vi "0x2 RIO-OCU command receive.vi"(11 "Manual Override Reader In":refnum<class "NetworkStreamReader.lvclass">) -> (3 "Manual Override Reader Out":refnum<class "NetworkStreamReader.lvclass">)   [LabVIEW 2011]
doc: "Gets commands from the OCU and sends them out to the rest of the code on the RIO using the globals."
uses:
  0x2 Classes/NetworkStreams/Reader/NetworkStreamReader.lvclass
  0x2 Typedefs/ocuCommands.ctl
  0x2 Typedefs/manual override.ctl
  2-Think/2 Typedefs/setpoints to boat.ctl
  2-Think/2 Typedefs/sail setpt.ctl
  2-Think/2 Typedefs/rudder angle.ctl
  0x2 Typedefs/ocuMessage.ctl
  2-Think/2 Classes/Waypoint/Waypoint.lvclass
  2-Think/2 Typedefs/UTM Circle.ctl
  2-Think/2 Classes/Missions/GenericMission/GenericMission.lvclass
  0x2 Typedefs/Current Waypoint.ctl
  0x2 Typedefs/Control values.ctl
  2-Think/2 Typedefs/Goodness Weightings.ctl
  2-Think/2 Typedefs/PI Constants.ctl
  2-Think/2 Typedefs/Apparent Wind Mode.ctl
  0x2 Typedefs/Sail Setting Tuning.ctl
  2-Think/2 Globals/2 Global.vi
  2-Think/2 Globals/2 TuningConstants.vi
  2-Think/2 Globals/2 Message Logger.vi
  2-Think/2 Classes/MissionQueue/MissionQueue.lvclass
  2-Think/2 Classes/Logger/Logger.lvclass
panel:
  out "Latest OCU Command":T1
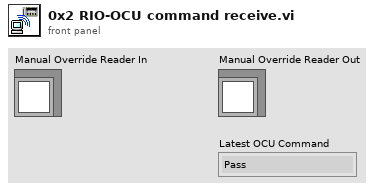
[diagram p1: front panel]
types:
  T1 = typedef "ocuCommands.ctl" = enum16{"Pass", "Send override", "Add waypoint", "Set waypoint number", "Stop", "Add Mission", "Reset Missions/Waypts", "Edit Control Values", "Add Global No-Sail", "Log Message"}
  T2 = typedef "manual override.ctl" = cluster{"Override Active Rudder":bool, "Setpoints":T3, "Override Active Sail":bool}
  T3 = typedef "setpoints to boat.ctl" = cluster{"Sail Position":T4, "Rudder Angle":T5}
  T4 = typedef "sail setpt.ctl" = dbl
  T5 = typedef "rudder angle.ctl" = dbl
  T6 = typedef "ocuMessage.ctl" = cluster{"OCU Command":T1, "Data":variant}
  T7 = typedef "UTM Circle.ctl" = cluster{"UTM Zone":dbl, "Hemisphere":enum16{"North", "South"}, "East":dbl, "North":dbl, "Radius":dbl}
  T8 = typedef "Current Waypoint.ctl" = i32
  T9 = typedef "Control values.ctl" = cluster{"Goodness Weightings":T10, "PI Constants":T11, "No Sail Zone\nTuning Quotient":dbl, "Heading Change Wind Adjustment":dbl, "Waypoint Tuning Quotient":dbl, "Apparent Wind Mode":T12, "RP Autonomous":bool, "Let Sail Out on Windcross":bool, "Shift Goal for currents":bool, "Round Buoy Safety":dbl, "Sail Setting Options":T13, "Defilter Wind Data":bool, "Irons Range":dbl, "Convincing Range":dbl, "Run Range":dbl, "Force tack attempt?":bool, "Minimum\ntack try\ntime?":dbl}
  T10 = typedef "Goodness Weightings.ctl" = cluster{"Target Importance":dbl, "No Sail Importance":dbl, "Change Importance":dbl, "Pure Waypoint \nImportance":dbl, "Pure Wind \nImportance":dbl}
  T11 = typedef "PI Constants.ctl" = cluster{"Proportional Gain":dbl, "Integral Time":dbl, "Derivative Time":dbl}
  T12 = typedef "Apparent Wind Mode.ctl" = cluster{"Desired Apparent\nWind Direction":dbl, "On":bool}
  T13 = typedef "Sail Setting Tuning.ctl" = cluster{"Linear\nMode":bool, "Sails Full In Point":dbl, "Sails Full Out Point":dbl}
  T14 = typedef "Waypoints List.ctl" = refnum<class "Waypoint.lvclass">[]
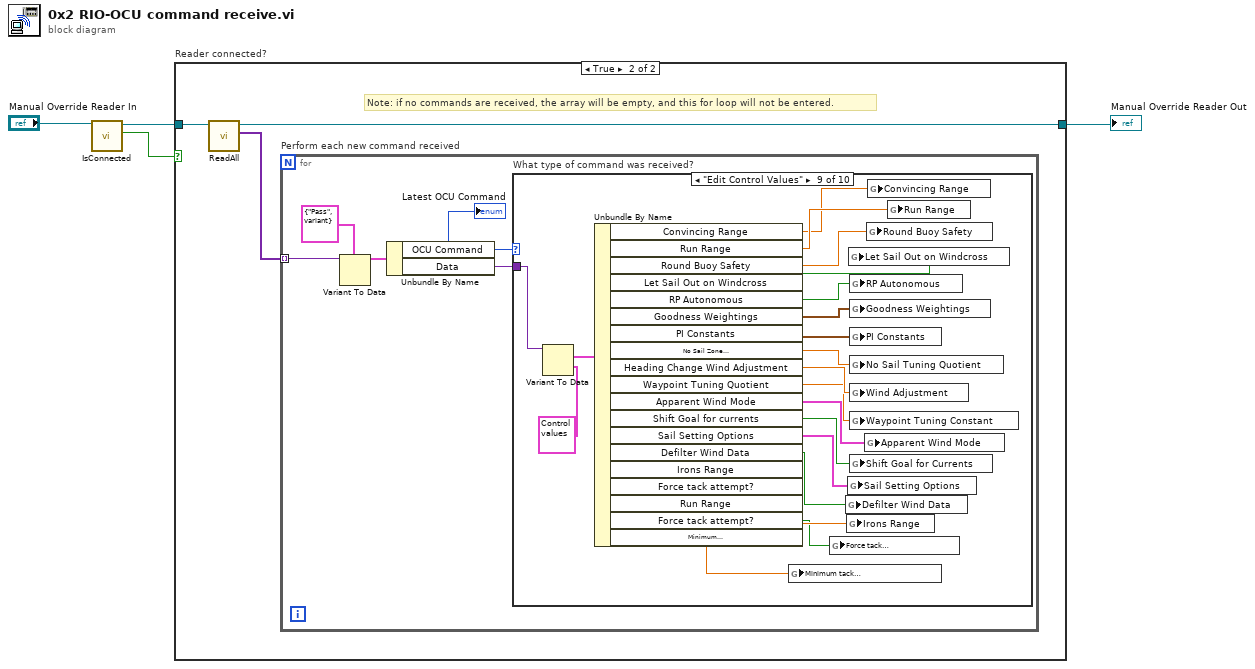
[diagram p0: block diagram]
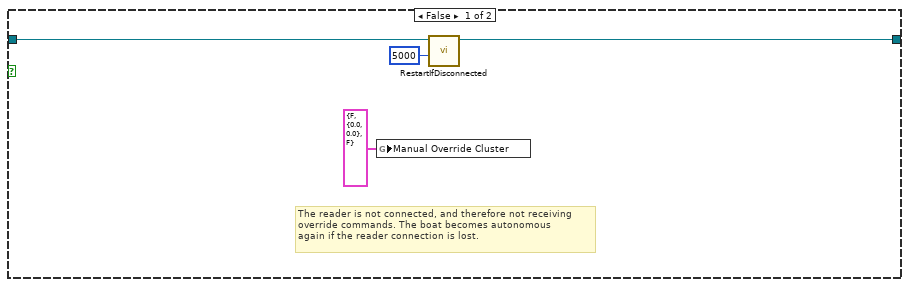
[diagram p2: hidden frame]
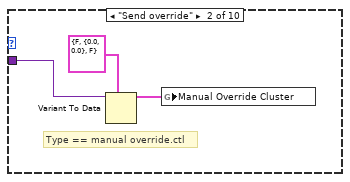
[diagram p4: hidden frame]
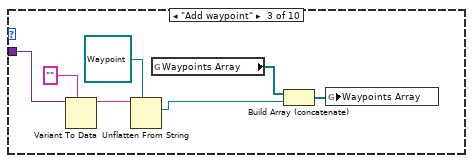
[diagram p5: hidden frame]
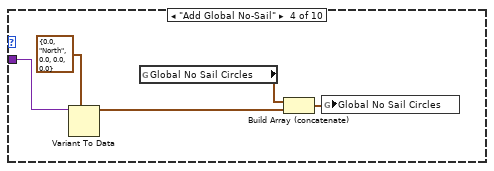
[diagram p6: hidden frame]
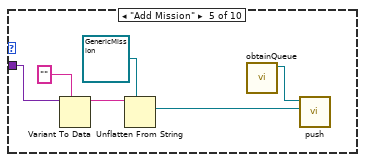
[diagram p7: hidden frame]
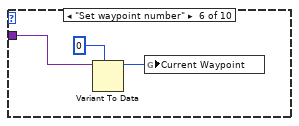
[diagram p8: hidden frame]
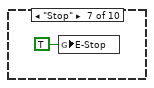
[diagram p9: hidden frame]
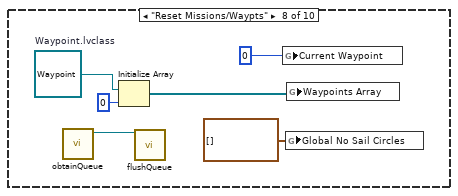
[diagram p10: hidden frame]
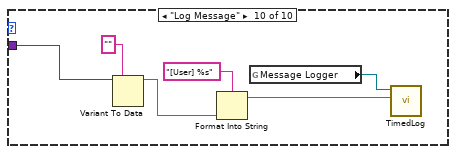
[diagram p11: hidden frame]
diagram:
  n1 = call "IsConnected.vi"("NetworkStreamReader in"="Manual Override Reader In") -> ("Connected?"=w3:bool, "NetworkStreamReader out"=w2:refnum<class "NetworkStreamReader.lvclass">)  [unwired: 8 in, 1 out]
  n2 = case "Reader connected?" shown="True" w3 {
    tunnel: w2 -> [w8 w10]
    tunnel: [w7 w9] -> w1
    frame False {
      # "The reader is not connected, and therefore not receiving\noverride commands. The boat becomes autonomous \nagain if the reader connection is lost."
      n3 = global write "2 Global.vi" "Manual Override Cluster"(T2 {"Override Active Rudder"=FALSE, "Setpoints"={"Sail Position"=0.0, "Rudder Angle"=0.0}, "Override Active Sail"=FALSE} ("Manual Override Cluster")) -> ()
      n4 = call "RestartIfDisconnected.vi"("connection timeout"=5000, "NetworkStreamReader in"=w8) -> ("NetworkStreamReader out"=w7:refnum<class "NetworkStreamReader.lvclass">)  [unwired: 8 in, 1 out]
    }
    frame True {
      # "Note: if no commands are received, the array will be empty, and this for loop will not be entered."
      n5 = call "ReadAll.vi"("NetworkStreamReader in"=w10) -> ("elements"=w11:variant[], "NetworkStreamReader out"=w9:refnum<class "NetworkStreamReader.lvclass">)  [unwired: 6 in, 3 out]
      n6 = for "Perform each new command received" {
        tunnel: w11 -> [w12] mode=indexing
        n7 = Variant To Data(type=T6 {"OCU Command"=enum."Pass", "Data"=variant} ("OCU Message"), Variant=w12) -> (data=w15:T6)  [unwired: 1 in, 1 out]
        n8 = Unbundle By Name(w15) -> ("OCU Command"=w14:T1, "Data"=w13:variant)
        "Latest OCU Command" <- w14
        n9 = case "What type of command was received?" shown="\"Edit Control Values\"" w14 {
          tunnel: w13 -> [_ w18 w26 w31 w35 w40 _ _ w67 w72]
          frame "Pass", Default {
          }
          frame "Send override" {
            # "Type == manual override.ctl"
            n10 = Variant To Data(type=T2 {"Override Active Rudder"=FALSE, "Setpoints"={"Sail Position"=0.0, "Rudder Angle"=0.0}, "Override Active Sail"=FALSE} ("Manual Override Cluster"), Variant=w18) -> (data=w17:T2)  [unwired: 1 in, 1 out]
            n11 = global write "2 Global.vi" "Manual Override Cluster"(w17) -> ()
          }
          frame "Add waypoint" {
            n12 = Variant To Data(type="", Variant=w26) -> (data=w22:string)  [unwired: 1 in, 1 out]
            n13 = Unflatten From String(type=refnum<class "Waypoint.lvclass"> refnum ("Waypoint.lvclass"), binary string=w22) -> (value=w20:refnum<class "Waypoint.lvclass">)  [unwired: 3 in, 2 out]
            n14 = global read "2 Global.vi" "Waypoints Array"() -> (w25:T14)
            n15 = Build Array (concatenate)(w25, w20) -> (w24:T14)
            n16 = global write "2 Global.vi" "Waypoints Array"(w24) -> ()
          }
          frame "Add Global No-Sail" {
            n17 = Variant To Data(type=T7 {"UTM Zone"=0.0, "Hemisphere"=enum."North", "East"=0.0, "North"=0.0, "Radius"=0.0} ("UTM Location"), Variant=w31) -> (data=w27:T7)  [unwired: 1 in, 1 out]
            n18 = global read "2 Global.vi" "Global No Sail Circles"() -> (w30:T7[])
            n19 = Build Array (concatenate)(w30, w27) -> (w29:T7[])
            n20 = global write "2 Global.vi" "Global No Sail Circles"(w29) -> ()
          }
          frame "Add Mission" {
            n21 = Variant To Data(type="", Variant=w35) -> (data=w36:string)  [unwired: 1 in, 1 out]
            n22 = Unflatten From String(type=refnum<class "GenericMission.lvclass"> refnum ("GenericMission.lvclass"), binary string=w36) -> (value=w32:refnum<class "GenericMission.lvclass">)  [unwired: 3 in, 2 out]
            n23 = call "obtainQueue.vi"() -> ("MissionQueue.lvclass"=w33:refnum<class "MissionQueue.lvclass">)  [unwired: 10 in, 1 out]
            n24 = call "push.vi"("GenericMission.lvclass"=w32, "MissionQueue in"=w33) -> ()  [unwired: 8 in, 2 out]
          }
          frame "Set waypoint number" {
            n25 = Variant To Data(type=T8 0 ("Current Waypoint"), Variant=w40) -> (data=w38:T8)  [unwired: 1 in, 1 out]
            n26 = global write "2 Global.vi" "Current Waypoint"(w38) -> ()
          }
          frame "Stop" {
            n27 = global write "2 Global.vi" "E-Stop"(TRUE ("E-Stop")) -> ()
          }
          frame "Reset Missions/Waypts" {
            w44 = refnum<class "Waypoint.lvclass"> refnum  # Waypoint.lvclass
            n28 = call "obtainQueue.vi"() -> ("MissionQueue.lvclass"=w43:refnum<class "MissionQueue.lvclass">)  [unwired: 10 in, 1 out]
            n29 = Initialize Array(w44, 0 ("dimension size")) -> (w46:refnum<class "Waypoint.lvclass">[])
            n30 = call "flushQueue.vi"("MissionQueue in"=w43) -> ()  [unwired: 8 in, 3 out]
            n31 = global write "2 Global.vi" "Current Waypoint"(T8 0 ("Current Waypoint")) -> ()
            n32 = global write "2 Global.vi" "Global No Sail Circles"(T7[] [] ("Global No Sail Circles")) -> ()
            n33 = global write "2 Global.vi" "Waypoints Array"(w46) -> ()
          }
          frame "Edit Control Values" {
            n34 = Variant To Data(type=T9 {"Goodness Weightings"={"Target Importance"=0.0, "No Sail Importance"=0.0, "Change Importance"=0.0, "Pure Waypoint \nImportance"=0.0, "Pure Wind \nImportance"=0.0}, "PI Constants"={"Proportional Gain"=0.0, "Integral Time"=0.0, "Derivative Time"=0.0}, "No Sail Zone\nTuning Quotient"=0.0, "Heading Change Wind Adjustment"=0.0, "Waypoint Tuning Quotient"=0.0, "Apparent Wind Mode"={"Desired Apparent\nWind Direction"=0.0, "On"=FALSE}, "RP Autonomous"=FALSE, "Let Sail Out on Windcross"=FALSE, "Shift Goal for currents"=FALSE, "Round Buoy Safety"=0.0, "Sail Setting Options"={"Linear\nMode"=FALSE, "Sails Full In Point"=0.0, "Sails Full Out Point"=0.0}, "Defilter Wind Data"=FALSE, "Irons Range"=0.0, "Convincing Range"=0.0, "Run Range"=0.0, "Force tack attempt?"=FALSE, "Minimum\ntack try\ntime?"=0.0}, Variant=w67) -> (data=w66:T9)  [unwired: 1 in, 1 out]
            n35 = Unbundle By Name(w66) -> ("Convincing Range"=w50:dbl, "Run Range"=w51:dbl, "Round Buoy Safety"=w55:dbl, "Let Sail Out on Windcross"=w57:bool, "RP Autonomous"=w58:bool, "Goodness Weightings"=w64:T10, "PI Constants"=w63:T11, "No Sail Zone\nTuning Quotient"=w65:dbl, "Heading Change Wind Adjustment"=w62:dbl, "Waypoint Tuning Quotient"=w61:dbl, "Apparent Wind Mode"=w59:T12, "Shift Goal for currents"=w56:bool, "Sail Setting Options"=w54:T13, "Defilter Wind Data"=w53:bool, "Irons Range"=w52:dbl, "Force tack attempt?"=w49:bool, "Minimum\ntack try\ntime?"=w48:dbl)  [unwired: 2 out]
            n36 = global write "2 TuningConstants.vi" "Minimum tack\ntry time?"(w48) -> ()
            n37 = global write "2 TuningConstants.vi" "Force tack\nattempt?"(w49) -> ()
            n38 = global write "2 Global.vi" "Defilter Wind Data"(w53) -> ()
            n39 = global write "2 TuningConstants.vi" "Irons Range"(w52) -> ()
            n40 = global write "2 TuningConstants.vi" "Sail Setting Options"(w54) -> ()
            n41 = global write "2 Global.vi" "Let Sail Out on Windcross"(w57) -> ()
            n42 = global write "2 Global.vi" "RP Autonomous"(w58) -> ()
            n43 = global write "2 TuningConstants.vi" "Goodness Weightings"(w64) -> ()
            n44 = global write "2 TuningConstants.vi" "PI Constants"(w63) -> ()
            n45 = global write "2 TuningConstants.vi" "No Sail Tuning Quotient"(w65) -> ()
            n46 = global write "2 TuningConstants.vi" "Wind Adjustment"(w62) -> ()
            n47 = global write "2 TuningConstants.vi" "Waypoint Tuning Constant"(w61) -> ()
            n48 = global write "2 Global.vi" "Shift Goal for Currents"(w56) -> ()
            n49 = global write "2 TuningConstants.vi" "Apparent Wind Mode"(w59) -> ()
            n50 = global write "2 Global.vi" "Round Buoy Safety"(w55) -> ()
            n51 = global write "2 Global.vi" "Convincing Range"(w50) -> ()
            n52 = global write "2 Global.vi" "Run Range"(w51) -> ()
          }
          frame "Log Message" {
            n53 = Variant To Data(type="" ("Message"), Variant=w72) -> (data=w69:string)  [unwired: 1 in, 1 out]
            n54 = Format Into String(format string="[User] %s", w69) -> (resulting string=w68:string)  [unwired: 2 in, 1 out]
            n55 = global read "2 Message Logger.vi" "Message Logger"() -> (w71:refnum<class "Logger.lvclass">)
            n56 = call "TimedLog.vi"("Message"=w68, "Logger in"=w71) -> ()  [unwired: 7 in, 3 out]
          }
        }
      }
    }
  }
  "Manual Override Reader Out" <- w1
